vi "Obtain Notifier.vi"(8 "error in (no error)":errorcluster, 11 "CVT_String in":refnum<class "CVT_String.lvclass">) -> (0 "error out":errorcluster, 3 "CVT_String out":refnum<class "CVT_String.lvclass">)   [LabVIEW 2024, in "Current Value Table.lvlib" / "CVT_String.lvclass"]
uses:
  CVT_String.lvclass
  CVT_String.lvclass/CVT_String.ctl
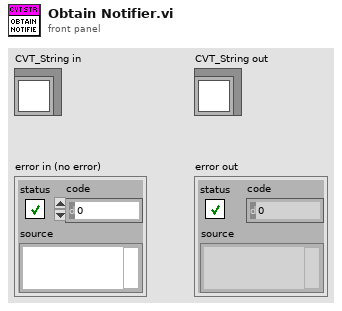
[diagram p1: front panel]
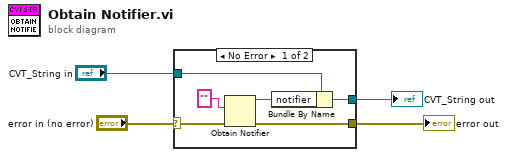
[diagram p0: block diagram]
diagram:
  n1 = case shown="No Error" "error in (no error)" {
    selector: "error in (no error)" -> [w8 w12]
    tunnel: [w7 w12] -> w3
    tunnel: [w6 w11] -> w1
    tunnel: "CVT_String in" -> [w10 w11]
    frame No Error {
      n2 = Obtain Notifier(notification data type="" ("element data type"), error in (no error)=w8) -> (notifier out=w9:refnum<notifier>, error out=w7:errorcluster)  [unwired: 2 in, 1 out]
      n3 = Bundle By Name(cluster=w10, "notifier"=w9) -> (w6:refnum<class "CVT_String.lvclass">)
    }
    frame Error {
    }
  }
  "error out" <- w3
  "CVT_String out" <- w1
